vi "Write Control Name.vi"(8 "error in (no error)":errorcluster, 10 "Control Name":string, 11 "Control Assertion in":refnum<class "Control Assertion.lvclass">) -> (0 "error out":errorcluster, 3 "Control Assertion out":refnum<class "Control Assertion.lvclass">)   [LabVIEW 2020, in "MacroAssert.lvlib" / "Control Assertion.lvclass"]
uses:
  Control Assertion.lvclass
  Control Assertion.lvclass/Control Assertion.ctl
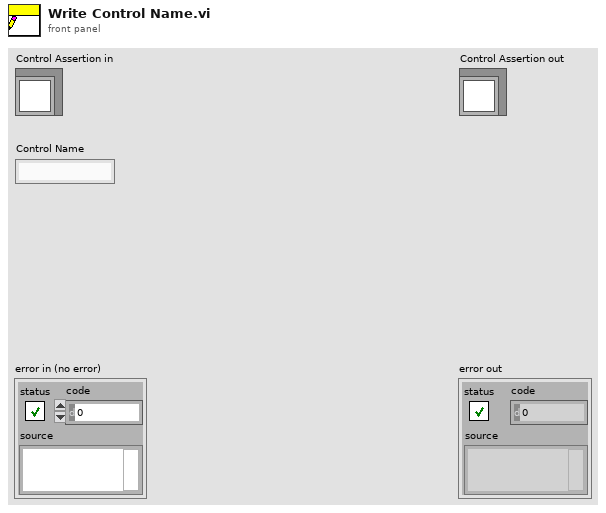
[diagram p1: front panel]
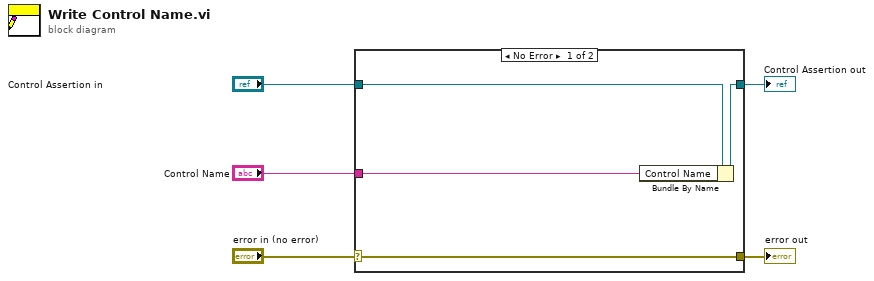
[diagram p0: block diagram]
diagram:
  n1 = case shown="No Error" "error in (no error)" {
    selector: "error in (no error)" -> [w9 w10]
    tunnel: [w9 w10] -> w4
    tunnel: [w7 w11] -> w2
    tunnel: "Control Assertion in" -> [w8 w11]
    tunnel: "Control Name" -> [w6 _]
    frame No Error {
      n2 = Bundle By Name(cluster=w8, "Control Name"=w6) -> (w7:refnum<class "Control Assertion.lvclass">)
    }
    frame Error {
    }
  }
  "error out" <- w4
  "Control Assertion out" <- w2
